vi "Detect Cans.vi"(11 "Image Dst Out":T1) -> ()   [LabVIEW 2014]
uses:
  <vilib>/vision/Image Controls.llb/IMAQ Image.ctl
  <vilib>/vision/NI_Vision_Development_Module.lvlib
panel:
  out "Image Out":T1
  in  "Search Rect":T2={"Left"=0, "Top"=0, "Right"=2147483647, "Bottom"=2147483647, "Rotation"=0.0} {"Rotation" format="%.2f"; "Left" scale=0.0..1024.0; "Right" scale=0.0..1024.0}
  out "Number of Matches":i32
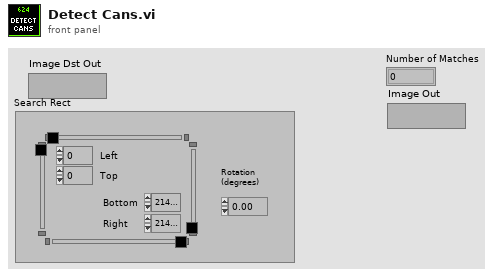
[diagram p1: front panel]
types:
  T1 = typedef "IMAQ Image.ctl" = refnum<image>
  T2 = typedef "IMAQ Rectangle" = cluster{"Left":i32, "Top":i32, "Right":i32, "Bottom":i32, "Rotation":dbl}
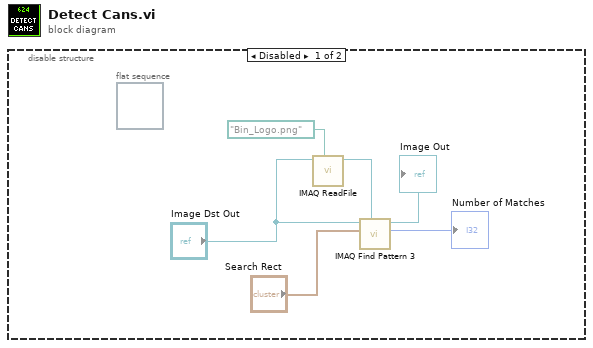
[diagram p0: block diagram]
diagram:
  n1 = disable-structure shown="Disabled" {
    frame Disabled {
      n2 = flat-sequence {
        frame #0 {
        }
      }
      n3 = call "IMAQ ReadFile"("File Path"=path "Bin_Logo.png", "Image"="Image Dst Out") -> ("Image Out"=w3:T1)  [unwired: 5 in, 4 out]
      n4 = call "IMAQ Find Pattern 3"("Template"=w3, "Search Rect"="Search Rect", "Image"="Image Dst Out") -> ("Number of Matches"=→"Number of Matches":i32, "Image Out"=→"Image Out":T1)  [unwired: 3 in, 4 out]
    }
    frame Enabled {
    }
  }
